vi "bias.vi"() -> ()   [LabVIEW 2025]
uses:
  <instrlib>/Keithley 2600 Series/Keithley 2600 Series.lvlib
panel:
  in  "source_range_gate":dbl(ring)=2.0 items=["200 mV"=0.2, "2 V"=2.0, "20 V"=20.0, "200 V"=200.0]
  in  "source_range_drain":dbl(ring)=2.0 items=["200 mV"=0.2, "2 V"=2.0, "20 V"=20.0, "200 V"=200.0]
  in  "range-gate":dbl(ring)=0.01 items=["100 nA"=1e-07, "1 uA"=1e-06, "10 uA"=1e-05, "100 uA"=0.0001, "1 mA"=0.001, "10 mA"=0.01, "100 mA"=0.1, "1 A"=1.0]
  in  "range-drain":dbl(ring)=0.01 items=["100 nA"=1e-07, "1 uA"=1e-06, "10 uA"=1e-05, "100 uA"=0.0001, "1 mA"=0.001, "10 mA"=0.01, "100 mA"=0.1, "1 A"=1.0]
  in  "file path (dialog if empty)":path
  out "range misurato":string
  out "range misurato":string
  in  "source autorange gate":bool
  in  "source autorange drain":bool
  in  "Range Mode (1: Auto Range On) 2":i32(ring)=1 items=["Auto Range Off", "Auto Range On", "Auto Range Follow Limit"]
  in  "Range Mode (1: Auto Range On)":i32(ring)=1 items=["Auto Range Off", "Auto Range On", "Auto Range Follow Limit"]
  in  "Source Function (1: Voltage) 2":i32(ring)=1 items=["Current", "Voltage"]
  in  "Source Function (1: Voltage)":i32(ring)=1 items=["Current", "Voltage"]
  in  "Autozero Mode (2: Autozero Auto) 2":i32(ring)=1 items=["Autozero Off", "Autozero Once", "Autozero Auto"]
  out "String 4":string
  out "String 3":string
  out "String 2":string
  out "String":string
  in  "inversione_porte":bool
  in  "Autozero Mode (2: Autozero Auto)":i32(ring)=1 items=["Autozero Off", "Autozero Once", "Autozero Auto"]
  in  "Periodo":ext(ring)=0.01 items=["500 uS", "1 mS", "2 mS", "5 mS", "10 mS", "20 mS", "50 mS", "100 mS", "200 mS", "500 mS", "1 S", "2 S", "5 S", "10 S", ""]
  out "finestra di misura":dbl
  out "measdelay":dbl
  in  "fattore-measdelay":i32=65
  out "Frequenza di rete (Hz)":dbl
  in  "Numero di punti":i32=11
  in  "llimit-gate":dbl=1.0 format="%#_13g"
  in  "limit-drain":dbl=1.0 format="%#_13g"
  in  "Tensione gate":dbl=1.0
  in  "Boolean":bool
  in  "tensione drain":dbl=1.0
  out "TEMPI":dbl[](array[numeric])
  out "TENSIONE":dbl[](array[numeric])
  out "CORRENTE":dbl[](array[numeric])
  out "TEMPI":dbl[](array[numeric])
  out "TENSIONE":dbl[](array[numeric])
  out "CORRENTE":dbl[](array[numeric])
  in  "stop 2":bool
  out "error out":errorcluster
  in  "stop":bool
  out "Firmware Revision":string
  out "Serial Number":string
  out "Model":string
  in  "VISA resource name":refnum<visa-resource-name>="USB0::0x05E6::0x2612::4671051::INSTR"
  # "Impostazioni funzione source"
  # "Impostazioni connessione"
  # "DRAIN"
  # "GATE"
  # "Auto Range Off"
  # "Auto Range On"
  # "Auto Range Off"
  # "Auto Range On"
  # "Impostazioni funzione misura"
  # "Impostazioni comuni"
  # "GATE"
  # "DRAIN"
  # "Auto Range Off"
  # "Auto Range On"
  # "Auto Range Off"
  # "Auto Range On"
  # "Controllo misura"
  # "tabella valori"
  # "SMUA"
  # "SMUB"
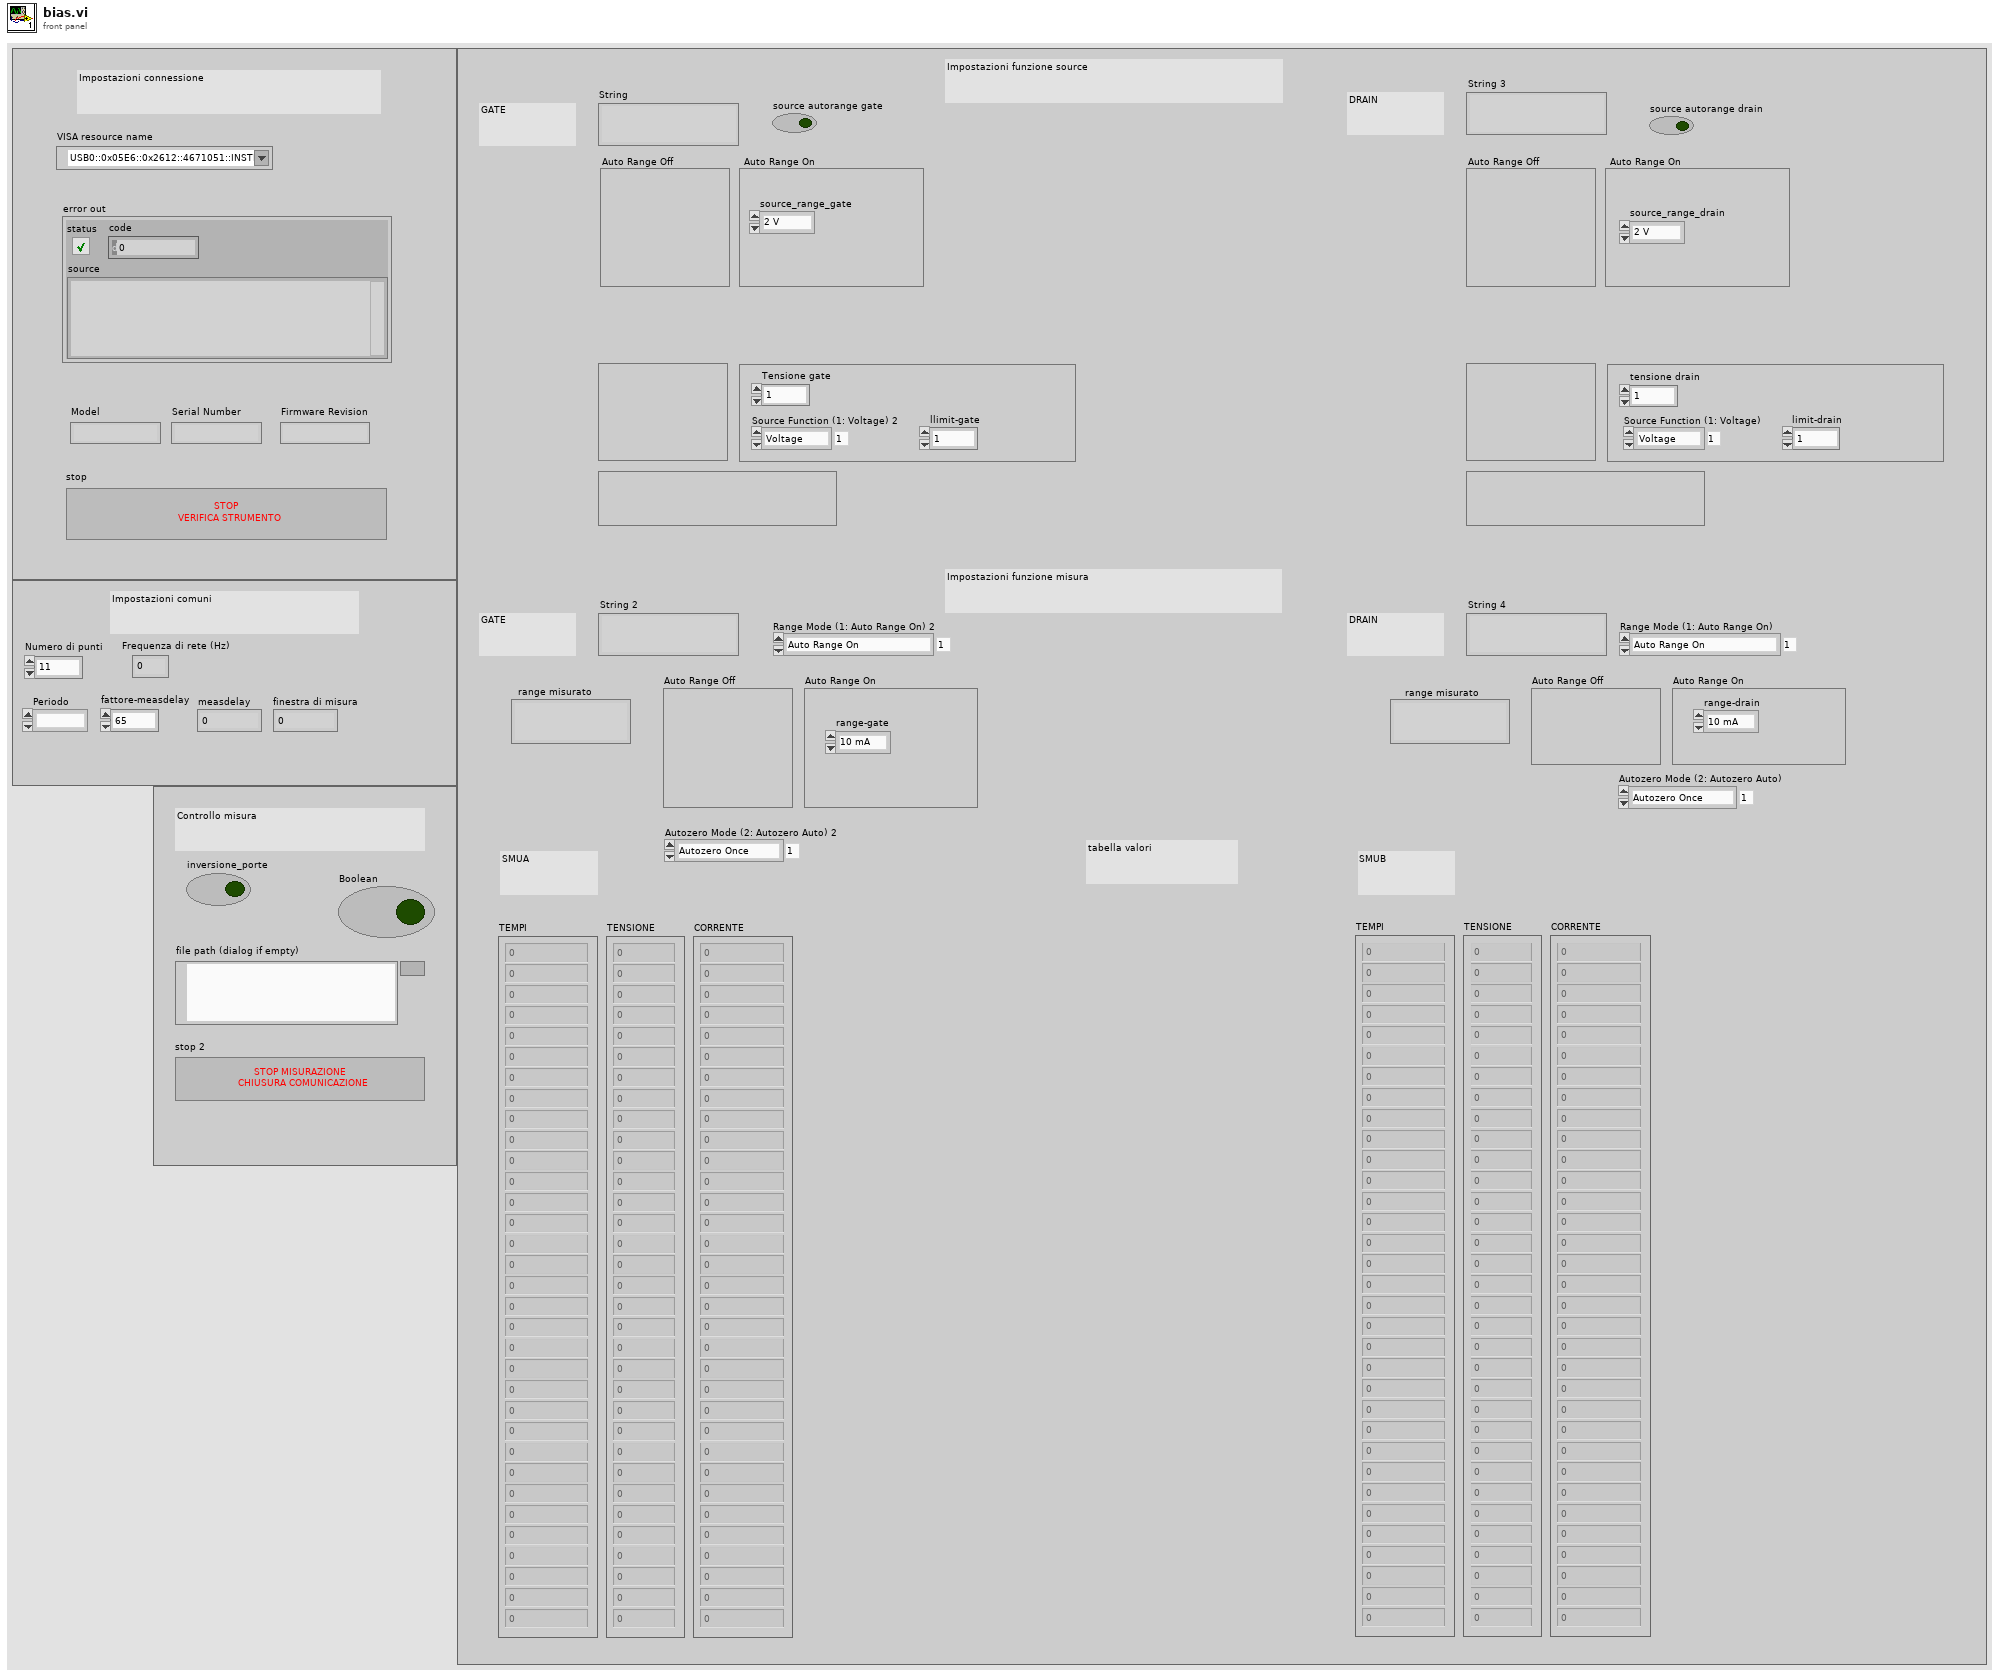
[diagram p1: front panel]
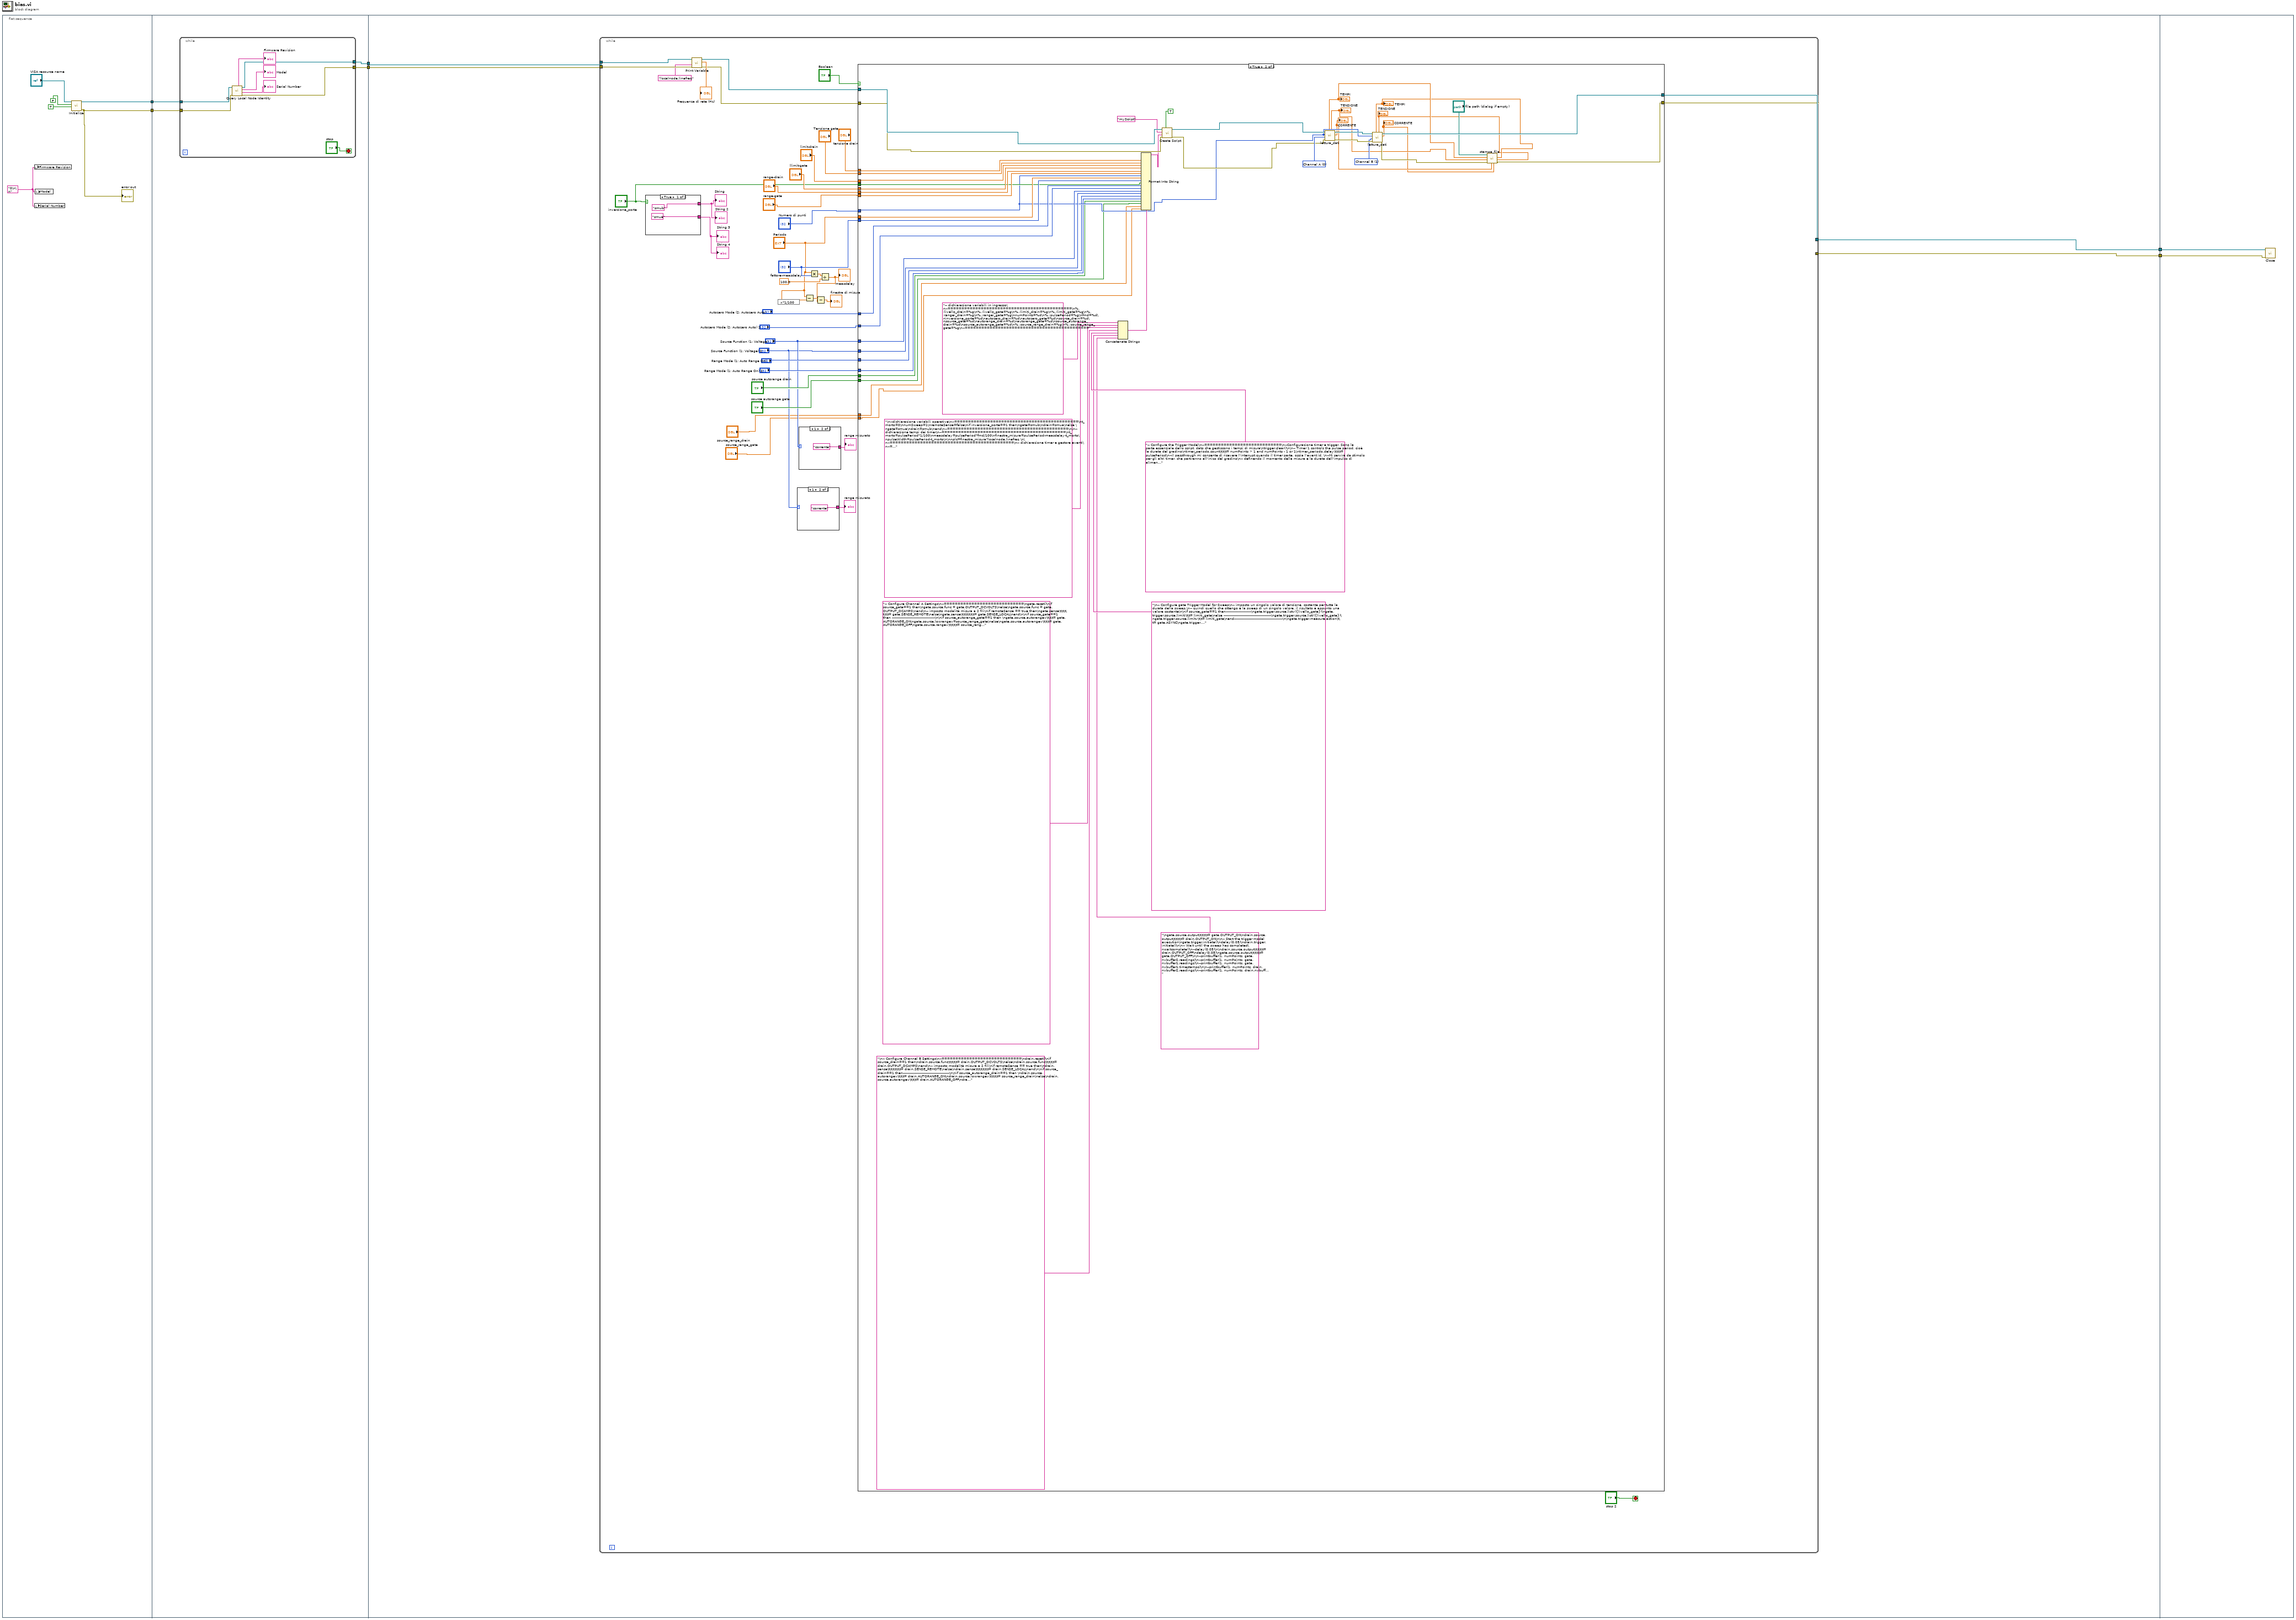
[diagram p0: block diagram]
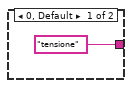
[diagram p2: hidden frame]
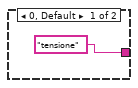
[diagram p3: hidden frame]
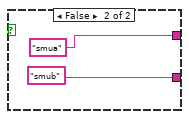
[diagram p4: hidden frame]
diagram:
  n1 = flat-sequence {
    tunnel: [w10] -> w5
    tunnel: [w9] -> w4
    tunnel: [w14] -> w6
    tunnel: w5 -> [w16]
    tunnel: w4 -> [w15]
    tunnel: [w13] -> w3
    tunnel: w6 -> [w28]
    tunnel: w3 -> [w27]
    tunnel: [w26] -> w2
    tunnel: [w25] -> w1
    tunnel: w2 -> [w129]
    tunnel: w1 -> [w128]
    frame #0 {
      w11 = "0\n\n"
      n2 = local write "Firmware Revision"(w11) -> ()
      n3 = local write "Serial Number"(w11) -> ()
      n4 = local write "Model"(w11) -> ()
      n5 = call <instrlib>:"Initialize.vi"("Reset (True)"=TRUE, "ID Query (True)"=FALSE, "VISA resource name"="VISA resource name") -> ("error out"=w9:errorcluster, "VISA resource name out"=w10:refnum<visa-resource-name>)  [unwired: 7 in]
      "error out" <- w9
    }
    frame #1 {
      n6 = while {
        tunnel: w16 -> [w20]
        tunnel: w15 -> [w19]
        tunnel: [w18] -> w14
        tunnel: [w17] -> w13
        stop <- "stop" stop-if-true
        n7 = call <instrlib>:"Query Local Node Identity.vi"("error in (no error)"=w19, "VISA resource name"=w20) -> ("error out"=w17:errorcluster, "Serial Number"=→"Serial Number":string, "Model"=→"Model":string, "VISA resource name out"=w18:refnum<visa-resource-name>, "Firmware Revision"=→"Firmware Revision":string)  [unwired: 5 in]
      }
    }
    frame #2 {
      n8 = while {
        tunnel: w28 -> [w58]
        tunnel: w27 -> [w57]
        tunnel: [w67] -> w26
        tunnel: [w66] -> w25
        stop <- "stop 2" stop-if-true
        n9 = case shown="True" "inversione_porte" {
          tunnel: ["smub" "smua"] -> w47
          tunnel: ["smua" "smub"] -> w46
          frame True {
          }
          frame False {
          }
        }
        "String" <- w47
        "String 2" <- w47
        "String 3" <- w46
        "String 4" <- w46
        n10 = call <instrlib>:"Print Variable.vi"("error in (no error)"=w57, "Variable Name"="localnode.linefreq", "VISA resource name"=w58) -> ("error out"=w42:errorcluster, "Number"=→"Frequenza di rete (Hz)":dbl, "VISA resource name out"=w41:refnum<visa-resource-name>)  [unwired: 5 in, 1 out]
        n11 = expression code="x*1/100"("Periodo") -> (w52:ext)
        n12 = case shown="1" "Source Function (1: Voltage) 2" {
          tunnel: ["tensione" "corrente"] -> w33
          frame 0, Default {
          }
          frame 1 {
          }
        }
        "range misurato" <- w33
        n13 = case shown="1" "Source Function (1: Voltage)" {
          tunnel: ["tensione" "corrente"] -> w34
          frame 0, Default {
          }
          frame 1 {
          }
        }
        "range misurato" <- w34
        n14 = Subtract(x="Periodo", y=w52) -> (x-y=w51:ext)
        n15 = Multiply(x="Periodo", y="fattore-measdelay") -> (x*y=w54:ext)
        n16 = Divide(x=w54, y=100.0) -> (x/y=w50:ext)
        "measdelay" <- w50
        n17 = Subtract(x=w51, y=w50) -> (x-y=→"finestra di misura":ext)
        n18 = case shown="True" "Boolean" {
          tunnel: [w78 w88] -> w67
          tunnel: [w77 w87] -> w66
          tunnel: w42 -> [w77 w125]
          tunnel: w41 -> [w78 w126]
          tunnel: "tensione drain" -> [_ w127]
          tunnel: "Numero di punti" -> [_ w95]
          tunnel: "llimit-gate" -> [_ w119]
          tunnel: "Tensione gate" -> [_ w121]
          tunnel: "limit-drain" -> [_ w120]
          tunnel: "range-drain" -> [_ w118]
          tunnel: "range-gate" -> [_ w117]
          tunnel: "Periodo" -> [_ w116]
          tunnel: "fattore-measdelay" -> [_ w115]
          tunnel: "inversione_porte" -> [_ w114]
          tunnel: "Autozero Mode (2: Autozero Auto)" -> [_ w113]
          tunnel: "Autozero Mode (2: Autozero Auto) 2" -> [_ w112]
          tunnel: "Source Function (1: Voltage)" -> [_ w111]
          tunnel: "Source Function (1: Voltage) 2" -> [_ w110]
          tunnel: "Range Mode (1: Auto Range On)" -> [_ w94]
          tunnel: "Range Mode (1: Auto Range On) 2" -> [_ w93]
          tunnel: "source autorange drain" -> [_ w92]
          tunnel: "source autorange gate" -> [_ w91]
          tunnel: "source_range_drain" -> [_ w90]
          tunnel: "source_range_gate" -> [_ w89]
          frame False {
          }
          frame True {
            w96 = 1 items=["Channel A", "Channel B"] ("Source Measure Unit Channel (0: Channel A)")
            w101 = 0 items=["Channel A", "Channel B"] ("Source Measure Unit Channel (0: Channel A)")
            n19 = Concatenate Strings("-- dichiarazione variabili in ingresso\n--=============================================\n%.;livello_drain=%g\n%.;livello_gate=%g\n%.;limiti_drain=%g\n%.;limiti_gate=%g\n%.;rangei_drain=%g\n%.;rangei_gate=%g\nnumPoints=%d\n%.;pulsePeriod=%g\nfmd=%d\ninversione_porte=%d\nautozero_drain=%d\nautozero_gate=%d\nsource_drain=%d\nsource_gate=%d\nautorange_drain=%d\nautorange_gate=%d\nsource_autorange_drain=%d\nsource_autorange_gate=%d\n%.;source_range_drain=%g\n%.;source_range_gate=%g\n--=============================================", "\n--dichiarazione variabili operative\n--=============================================\nt_morto=0\nnumSweep=1\nremoteSense=false\nif inversione_porte==1 then\ngate=smub\ndrain=smua\nelse \ngate=smua\ndrain=smub\nend\n--============================================\n\n-- dichiarazione tempi dei timer\n--=============================================\nt_morto=pulsePeriod*1/100\nmeasdelay=pulsePeriod*fmd/100\nfinestra_misura=pulsePeriod-measdelay-t_morto\npulseWidth=pulsePeriod-t_morto\n\nnplc=finestra_misura*localnode.linefreq \n\n--=============================================\n-- dichiarazione timer e gestore eventi\n--=============================================\n-- Timer 1: timer periodo (larghezza gradino)\ntimer_periodo=trigger.timer[1]\n-- Timer 2: Timer ritardo misura\ntimer_misura=trigger.timer[2]\n-- Timer 3: Pulse Width Timer\ntimer_larghezza_impulso=trigger.timer[3]\n\n-- Gestore eventi 1: Event Blender per la partenza di iniziale di gate e l'aggiornamento di gate al trigger di drain\ngestore_avvio_gate=trigger.blender[1]\n--=============================================", "-- Configure Channel A Settings\n--=============================\ngate.reset()\nif source_gate==1 then\ngate.source.func = gate.OUTPUT_DCVOLTS\nelse\ngate.source.func = gate.OUTPUT_DCAMPS\nend\n-- imposto modalità misura a 2 fili\nif remoteSense == true then\ngate.sense\t\t\t\t\t\t= gate.SENSE_REMOTE\nelse\ngate.sense\t\t\t\t\t\t= gate.SENSE_LOCAL\nend\n\nif source_gate==1 then ---------------------------------------\n\nif source_autorange_gate==1 then \ngate.source.autorangev\t\t\t= gate.AUTORANGE_ON\ngate.source.lowrangev=source_range_gate\nelse\ngate.source.autorangev\t\t\t= gate.AUTORANGE_OFF\ngate.source.rangev\t\t\t\t= source_range_gate\nend \n\ngate.source.levelv\t\t\t\t= 0\n-- Set the DC bias limit.  This is not the limit used during the pulses. ma è il valore di idle della gate\ngate.source.limiti\t\t\t\t= limiti_gate\n\nelse------------------------\n\nif source_autorange_gate==1 then\ngate.source.autorangei\t\t\t= gate.AUTORANGE_ON\ngate.source.lowrangei=source_range_gate\nelse\ngate.source.autorangei\t\t\t= gate.AUTORANGE_OFF\ngate.source.rangei\t\t\t= source_range_gate\nend\n\ngate.source.leveli\t\t\t\t= 0\n-- Set the DC bias limit.  This is not the limit used during the pulses. ma è il valore di idle della gate\ngate.source.limitv\t\t\t\t= limiti_gate\nend --------------------------------------------------\n\n\n-- Disabling Auto-Ranging and Auto-Zero ensures accurate and consistent timing\n\nif autozero_gate==0 then\ngate.measure.autozero\t\t\t= gate.AUTOZERO_OFF\nelseif autozero_gate==1 then\ngate.measure.autozero\t\t\t= gate.AUTOZERO_ONCE\nelse\ngate.measure.autozero\t\t\t= gate.AUTOZERO_AUTO\nend\n\nif autorange_gate==0 then ------------------------\n\nif source_gate==1 then\ngate.measure.autorangei\t\t\t= gate.AUTORANGE_OFF\ngate.measure.rangei\t\t\t\t= rangei_gate\nelse\ngate.measure.autorangev\t\t\t= gate.AUTORANGE_OFF\ngate.measure.rangev\t\t\t\t= rangei_gate\nend\n\nelseif  autorange_gate==1 then -----------\n\nif source_gate==1 then\ngate.measure.autorangei\t\t\t= gate.AUTORANGE_ON\ngate.measure.lowrangei\t\t\t\t= rangei_gate\nelse\ngate.measure.autorangev\t\t\t= gate.AUTORANGE_ON\ngate.measure.lowrangev\t\t\t\t= rangei_gate\nend\n\nelse --------------------------\n\nend -------------------------------\n\ngate.measure.nplc\t\t\t\t= nplc\n-- A timer will be used to set the measure delay and synchronize the measurement\n-- between the two SMUs so set the built in delay to 0.\ngate.measure.delay\t\t\t\t= 0\n\n-- Prepare the Reading Buffers\ngate.nvbuffer1.clear()\ngate.nvbuffer1.collecttimestamps= 1\ngate.nvbuffer2.clear()\ngate.nvbuffer2.collecttimestamps = 1\n--=============================\n-- End Channel A Settings\n", "\n-- Configure Channel B Settings\n--=============================\ndrain.reset()\nif source_drain==1 then\ndrain.source.func\t\t\t\t= drain.OUTPUT_DCVOLTS\nelse\ndrain.source.func\t\t\t\t= drain.OUTPUT_DCAMPS\nend\n-- imposto modalità misura a 2 fili\nif remoteSense == true then\ndrain.sense\t\t\t\t\t\t= drain.SENSE_REMOTE\nelse\ndrain.sense\t\t\t\t\t\t= drain.SENSE_LOCAL\nend\n\nif source_drain==1 then------------------------------------------\n\nif source_autorange_drain==1 then \ndrain.source.autorangev\t\t\t= drain.AUTORANGE_ON\ndrain.source.lowrangev\t\t\t\t= source_range_drain\nelse\ndrain.source.autorangev\t\t\t= drain.AUTORANGE_OFF\ndrain.source.rangev\t\t\t\t=source_range_drain\nend\n\ndrain.source.levelv\t\t\t\t= 0\n-- Set the DC bias limit.  This is not the limit used during the pulses. ma è il valore di idle della smu\ndrain.source.limiti\t\t\t\t= limiti_drain\nelse----------------------------------------------------\nif source_autorange_drain==1 then \ndrain.source.autorangei\t\t\t= drain.AUTORANGE_ON\ndrain.source.lowrangei\t\t\t\t=source_range_drain\nelse\ndrain.source.autorangei\t\t\t= drain.AUTORANGE_OFF\ndrain.source.rangei\t\t\t\t=source_range_drain\nend\ndrain.source.leveli\t\t\t\t= 0\n-- Set the DC bias limit.  This is not the limit used during the pulses. ma è il valore di idle della smu\ndrain.source.limitv\t\t\t\t= limiti_drain\nend----------------------------------------------\n\n-- Disabling Auto-Ranging and Auto-Zero ensures accurate and consistent timing\n\nif autozero_drain==0 then\ndrain.measure.autozero\t\t\t= drain.AUTOZERO_OFF\nelseif autozero_drain==1 then\ndrain.measure.autozero\t\t\t= drain.AUTOZERO_ONCE\nelseif autozero_drain==2 then\ndrain.measure.autozero\t\t\t= drain.AUTOZERO_AUTO\nend\n\nif autorange_drain==0 then --------------------------------\n\nif source_drain==1 then\ndrain.measure.autorangei\t\t\t= drain.AUTORANGE_OFF\ndrain.measure.rangei\t\t\t\t= rangei_drain\nelse\ndrain.measure.autorangev\t\t\t= drain.AUTORANGE_OFF\ndrain.measure.rangev\t\t\t\t= rangei_drain\nend\n\n\n\nelseif  autorange_drain==1 then ----------------------------\n\nif source_drain==1 then\ndrain.measure.autorangei\t\t\t= drain.AUTORANGE_ON\ndrain.measure.lowrangei\t\t\t\t= rangei_drain\nelse\ndrain.measure.autorangev\t\t\t= drain.AUTORANGE_ON\ndrain.measure.lowrangev\t\t\t\t= rangei_drain\nend\n\nelse\n\nend --------------------------------------------------------------\n\ndrain.measure.nplc\t\t\t\t= nplc\n-- A timer will be used to set the measure delay and synchronize the measurement\n-- between the two SMUs so set the built in delay to 0.\ndrain.measure.delay\t\t\t\t= 0\n\n-- Prepare the Reading Buffers\ndrain.nvbuffer1.clear()\ndrain.nvbuffer1.collecttimestamps= 1\ndrain.nvbuffer2.clear()\ndrain.nvbuffer2.collecttimestamps= 1\n--=============================\n-- End Channel B Settings", "-- Configure the Trigger Model\n--============================\n--Configurazione timer e trigger. Sono la parte essenziale dello script, dato che gestiscono i tempi di misura\ntrigger.clear()\n\n-- Timer 1 controls the pulse period, cioè la durata del gradino\ntimer_periodo.count\t\t\t= numPoints > 1 and numPoints - 1 or 1\ntimer_periodo.delay\t\t\t= pulsePeriod\n--il passthrough mi consente di ricevere l'interrupt quando il timer parte, ossia l'event id. \n--Mi servirà da stimolo per gli altri timer, che partiranno all'inizo del gradino\n-- definendo il momento della misura e la durata dell'impulso di alimentazione\ntimer_periodo.passthrough\t= true\n-- il timer 1 parte quando la drain, in questo caso, inizia la sweep: cioè entra nello stato armed\ntimer_periodo.stimulus\t\t= drain.trigger.ARMED_EVENT_ID \n\n-- Timer 2 controls the measurement. il timer 2 gestisce il ritardo di misura. scaduto quello, inizia la finestra di misura\ntimer_misura.count\t\t\t= 1\ntimer_misura.delay\t\t\t= measdelay\n-- il passthrough è false perchè l'interrupt lo produrre alla fine. \n-- Scaduto il delay di misura, inizia la finestra di misura\ntimer_misura.passthrough\t= false\n--il timer 1 grazie al passthrough mi fa partire il timer 2 all'inizio del gradino\ntimer_misura.stimulus\t\t= timer_periodo.EVENT_ID \n\n-- Timer 3 controls the pulse width\ntimer_larghezza_impulso.count\t\t\t= 1\ntimer_larghezza_impulso.delay\t\t\t= pulseWidth\n-- il passthrough è false perchè l'interrupt me lo produce alla fine, perchè \ntimer_larghezza_impulso.passthrough\t= false\n--il timer 1 grazie al passthrough mi fa partire il timer 3 all'inizio del gradino\ntimer_larghezza_impulso.stimulus\t\t= timer_periodo.EVENT_ID", "\n-- Configure gate Trigger Model for Sweep\n-- imposto un singolo valore di tensione, costante per tutta la durata della sweep.\n-- quindi quello che ottengo è la sweep di un singolo valore. il risultato è appunto una valore costante\n\nif source_gate==1 then-----------------------\ngate.trigger.source.listv({livello_gate})\ngate.trigger.source.limiti\t\t= limiti_gate\nelse -------------------------------------------\ngate.trigger.source.listi({livello_gate})\ngate.trigger.source.limitv\t\t= limiti_gate\nend--------------------------------------------\n\ngate.trigger.measure.action\t\t= gate.ASYNC\ngate.trigger.measure.iv(gate.nvbuffer1, gate.nvbuffer2)\n--fine impulso: se voglio una dc sweep, anzichè mandare in idle l'uscita, la tengo costante\ngate.trigger.endpulse.action\t= gate.SOURCE_HOLD\n-- endsweep mi dice cosa fare quando finisce l'operazione sweep\ngate.trigger.endsweep.action\t= gate.SOURCE_HOLD\ngate.trigger.arm.count = 1\ngate.trigger.count\t\t\t\t= numSweep\n-- arm sweep indica quanto sweep deve fare \ndrain.trigger.arm.stimulus\t\t= 0\n\n\n--event blender per la partenza\ngestore_avvio_gate.orenable = true\ngestore_avvio_gate.stimulus[1] = gate.trigger.ARMED_EVENT_ID\ngestore_avvio_gate.stimulus[2] = drain.trigger.ARMED_EVENT_ID \n\n--dico quali stimoli/timer attivano le azioni\ngate.trigger.source.stimulus = gestore_avvio_gate.EVENT_ID \ngate.trigger.measure.stimulus\t= timer_misura.EVENT_ID\ngate.trigger.endpulse.stimulus\t= drain.trigger.SWEEP_COMPLETE_EVENT_ID\n\ngate.trigger.source.action\t\t= gate.ENABLE\n\n-- Configure drain Trigger Model for Sweep\nif source_drain==1 then------------------------\ndrain.trigger.source.listv({livello_drain})\ndrain.trigger.source.limiti\t\t= limiti_drain\nelse---------------------------------------------\ndrain.trigger.source.listi({livello_drain})\ndrain.trigger.source.limitv\t\t= limiti_drain\nend---------------------------------------------\n\ndrain.trigger.measure.action\t\t= drain.ENABLE\ndrain.trigger.measure.iv(drain.nvbuffer1, drain.nvbuffer2)\n--fine impulso: se voglio una dc sweep, anzichè mandare in idle l'uscita, la tengo costante\ndrain.trigger.endpulse.action\t= drain.SOURCE_HOLD\n-- endsweep mi dice cosa fare quando finisce l'operazione sweep\ndrain.trigger.endsweep.action\t= drain.SOURCE_HOLD\ndrain.trigger.arm.count = numSweep\n-- num punti sweep\ndrain.trigger.count\t\t\t\t= numPoints\n-- arm sweep indica quanto sweep deve fare\ndrain.trigger.arm.stimulus\t\t= 0\n--dico quali timer attivanzo le azioni\ndrain.trigger.source.stimulus\t= timer_periodo.EVENT_ID\ndrain.trigger.measure.stimulus\t= timer_misura.EVENT_ID\ndrain.trigger.endpulse.stimulus\t= timer_larghezza_impulso.EVENT_ID\ndrain.trigger.source.action\t\t= drain.ENABLE\n--==============================\n-- End Trigger Model Configuration", "\ngate.source.output\t\t\t\t= gate.OUTPUT_ON\ndrain.source.output\t\t\t\t= drain.OUTPUT_ON\n\n-- Start the trigger model execution\ngate.trigger.initiate()\ndelay(0.05)\ndrain.trigger.initiate()\n\n-- Wait until the sweep has completed\nwaitcomplete()\n--delay(0.05)\n\ndrain.source.output\t\t\t\t= drain.OUTPUT_OFF\ndelay(0.05)\ngate.source.output\t\t\t\t= gate.OUTPUT_OFF\n\n--printbuffer(1, numPoints, gate.nvbuffer2.readings)\n--printbuffer(1, numPoints, gate.nvbuffer1.readings)\n--printbuffer(1, numPoints, gate.nvbuffer1.timestamps)\n\n--printbuffer(1, numPoints, drain.nvbuffer2.readings)\n--printbuffer(1, numPoints, drain.nvbuffer1.readings)\n--printbuffer(1, numPoints, drain.nvbuffer1.timestamps)") -> (w109:string)
            n20 = Format Into String(format string=w109, w127, w121, w120, w119, w118, w117, w95, w116, w115, w114, w113, w112, w111, w110, w94, w93, w92, w91, w90, w89) -> (resulting string=w124:string)  [unwired: 2 in, 1 out]
            n21 = call <instrlib>:"Create Script.vi"("Auto Run (F: Disable)"=TRUE, "error in (no error)"=w125, "Source Code"=w124, "Script Variable"="myScript", "VISA resource name"=w126) -> ("error out"=w99:errorcluster, "VISA resource name out"=w100:refnum<visa-resource-name>)  [unwired: 5 in]
            n22 = call "lettura_dati.vi"("error in (no error)"=w99, "Source Measure Unit Channel (0: Channel A)"=w101, "End Index (1)"=w95, "VISA resource name"=w100) -> ("error out"=w98:errorcluster, "CORRENTE"=w82:dbl[], "VISA resource name out"=w97:refnum<visa-resource-name>, "TENSIONE"=w83:dbl[], "TEMPI"=w84:dbl[])  [unwired: 3 in]
            "CORRENTE" <- w82
            "TEMPI" <- w84
            "TENSIONE" <- w83
            n23 = call "lettura_dati.vi"("error in (no error)"=w98, "Source Measure Unit Channel (0: Channel A)"=w96, "End Index (1)"=w95, "VISA resource name"=w97) -> ("error out"=w86:errorcluster, "CORRENTE"=w79:dbl[], "VISA resource name out"=w88:refnum<visa-resource-name>, "TENSIONE"=w80:dbl[], "TEMPI"=w81:dbl[])  [unwired: 3 in]
            "TEMPI" <- w81
            "TENSIONE" <- w80
            "CORRENTE" <- w79
            n24 = call "stampa_file.vi"(1:"Tensione"=w80, 2:"Tempo"=w81, 4:"Corrente"=w79, 6:"Corrente"=w82, "error in (no error)"=w86, 9:"Tensione"=w83, 10:"Tempo"=w84, "file path (dialog if empty)"="file path (dialog if empty)") -> ("error out"=w87:errorcluster)  [unwired: 2 in, 1 out]
          }
        }
      }
    }
    frame #3 {
      n25 = call <instrlib>:"Close.vi"("error in (no error)"=w128, "VISA resource name"=w129) -> ()  [unwired: 9 in, 1 out]
    }
  }
